vi "HapticSPM_force_bonding.vi"() -> ()   [LabVIEW 2023]
uses:
  Haptic-Programming-Interface/LabVIEW VIs/Haptic Prog Interface/Haptic Prog Interface.lvlib
panel:
  out "k":dbl format="%#_13g"
  out "Setpoint":dbl format="%#_13g"
  out "Force Function":string
  in  "Input Function":i32 min=0 max=4 step=1
  out "Potential vs Distance":cluster{dbl[], dbl[]}(graph)
  out "Force vs Distance":cluster{dbl[], dbl[]}(graph)
  out "Z-Position (pm)":dbl caption="Numeric" min=0.0 format="%#.1p"
  out "Force":dbl(knob) scale=-4.0..4.0
  in  "Gain":dbl=1.0 caption="Numeric" format="%.1g"
  # "Super Ultra Mega Haptic SPM Controller 3000"
  # "Height"
  # "Move pen in all three dimensions to calibrate before feeling surface\n\nClick \"ENTER\" to turn off recommended settings\n\nChange \"Setpoint\" and \"k\" parameters to adjust the feel of the force\n\nUse the \"PAGE UP\" or \"PAGE DOWN\" key to change the force function\n\nHold the pen as high as possible before changing force functions"
  # "Force"
  # "create bonding picture on this mod"
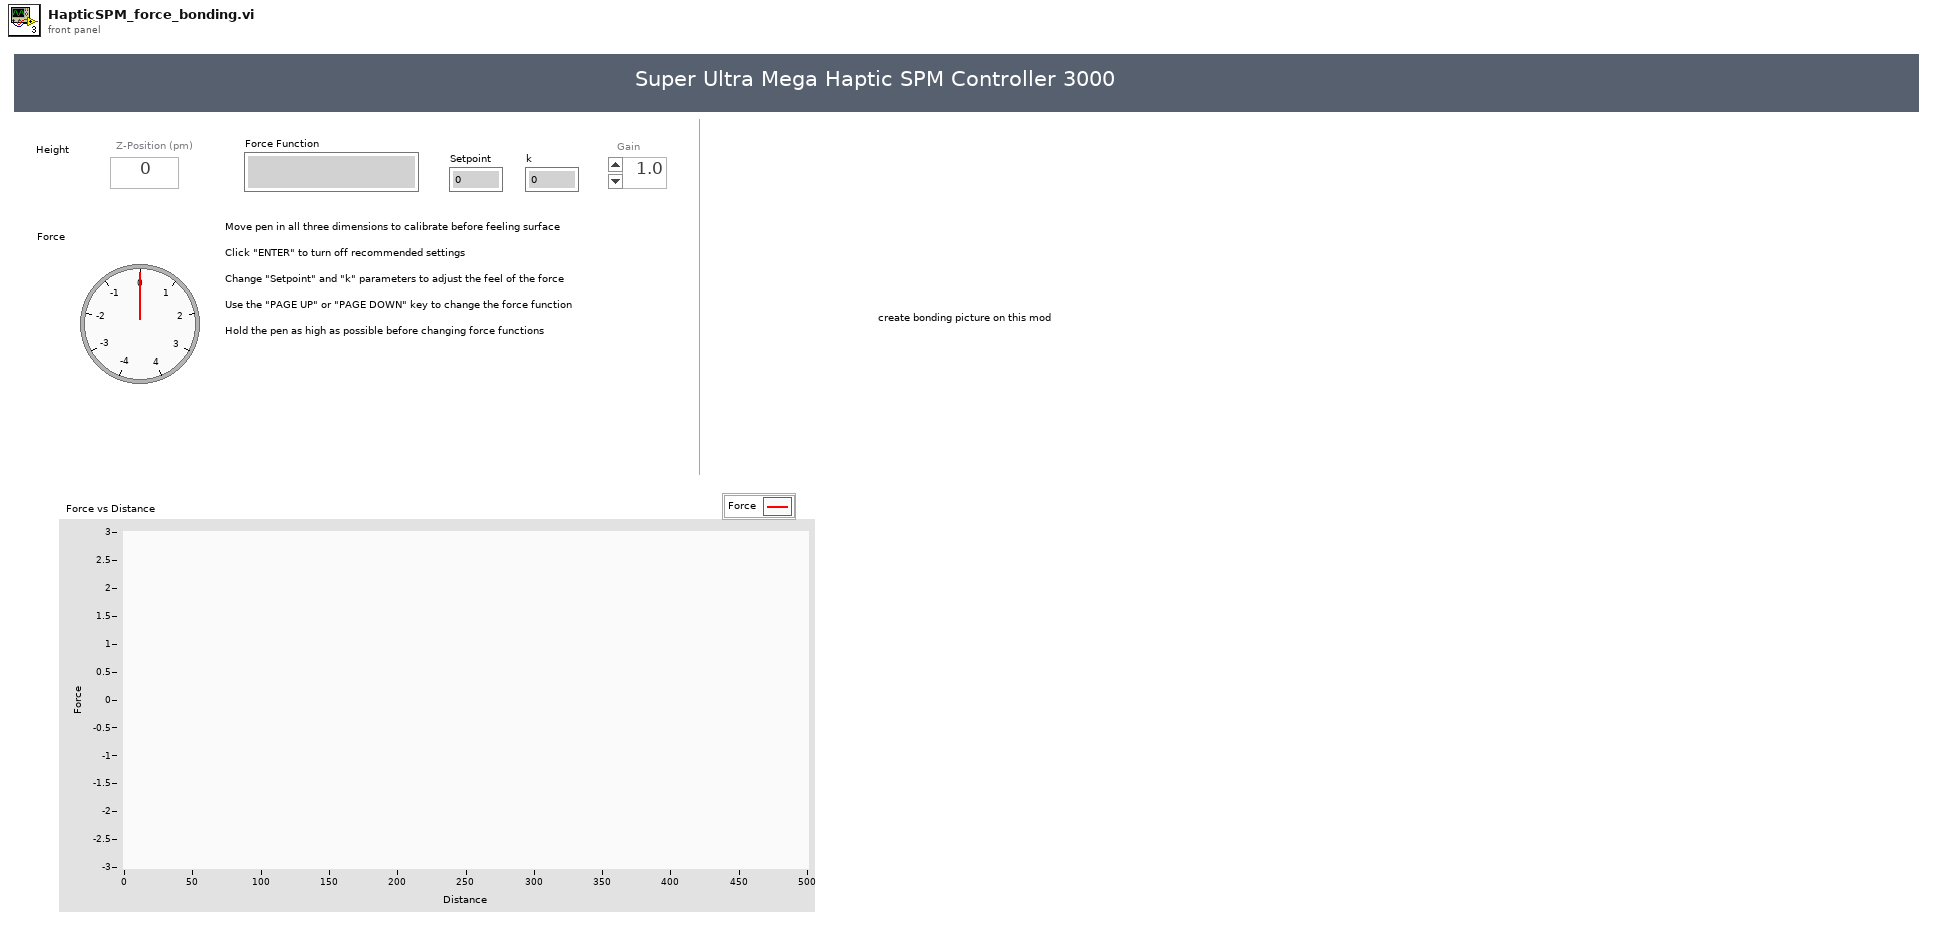
[diagram p1: front panel]
types:
  T1 = cluster{"Fx (N)":dbl, "Fy (N)":dbl, "Fz (N)":dbl}
  T2 = cluster{"kx (N/m)":dbl, "ky (N/m)":dbl, "kz (N/m)":dbl}
  T3 = cluster{"X Drag":bool, "Y Drag":bool, "Z Drag":bool}
  T4 = cluster{"x (mm)":dbl, "y (mm)":dbl, "z (mm)":dbl}
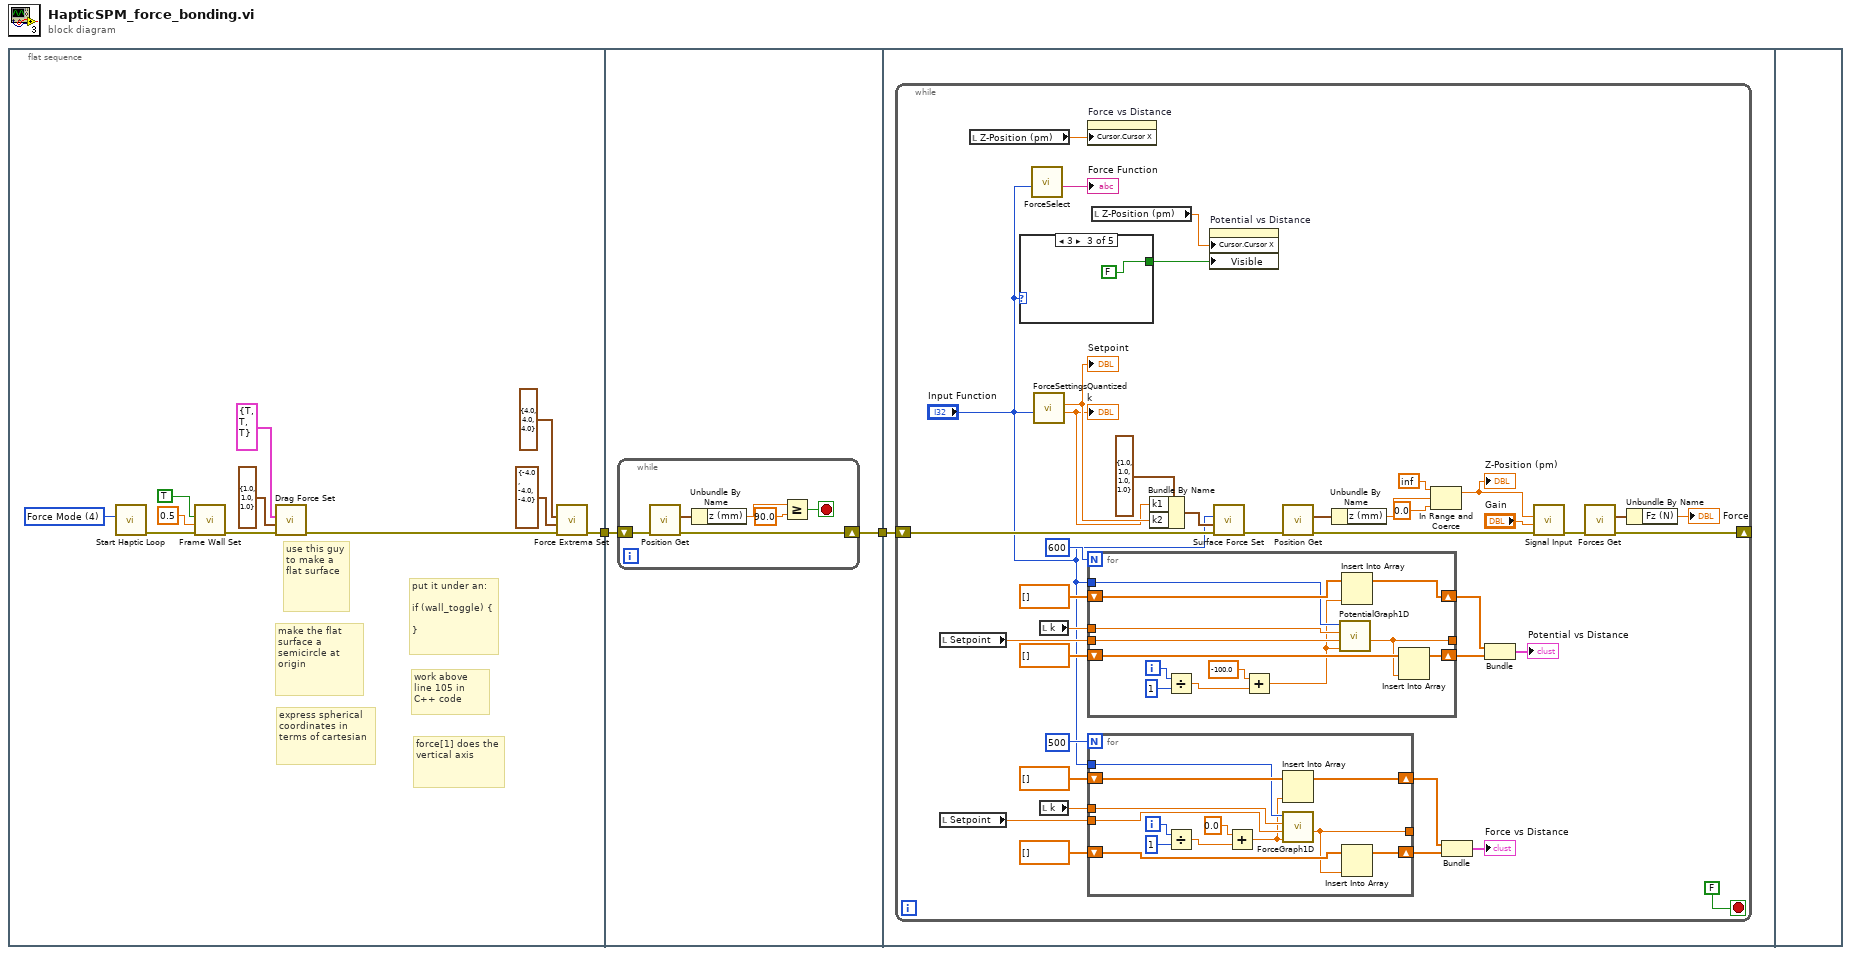
[diagram p0: block diagram]
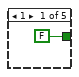
[diagram p2: hidden frame]
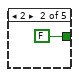
[diagram p3: hidden frame]
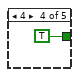
[diagram p4: hidden frame]
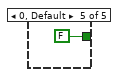
[diagram p5: hidden frame]
diagram:
  n1 = flat-sequence {
    tunnel: [w11] -> w2
    tunnel: w2 -> [w15]
    tunnel: [w14] -> w1
    tunnel: w1 -> [w22]
    frame #0 {
      w13 = u16 4 items=["Custom Mode", "Read Mode", "Write Mode", "Position Mode", "Force Mode"] ("Mode Selection")
      # "force[1] does the vertical axis"
      # "put it under an:\n\nif (wall_toggle) {\n\n}"
      # "work above line 105 in C++ code"
      # "express spherical coordinates in terms of cartesian"
      # "make the flat surface a semicircle at origin"
      # "use this guy to make a flat surface"
      n2 = call "Start Haptic Loop.vi"("Mode Selection"=w13) -> ("error out"=w4:errorcluster)  [unwired: 10 in]
      n3 = call "Frame Wall Set.vi"("error in (no error)"=w4, "Wall Stiffness (N/m)"=0.5 ("Wall Stiffness"), "Restrict to Frame"=TRUE) -> ("error out"=w3:errorcluster)  [unwired: 8 in]
      n4 = call "Drag Force Set.vi"("error in (no error)"=w3, "Drag Coefficients (N/m)"=T2 {"kx (N/m)"=1.0, "ky (N/m)"=1.0, "kz (N/m)"=1.0} ("Drag Coefficients"), "Drag Force Toggles"=T3 {"X Drag"=TRUE, "Y Drag"=TRUE, "Z Drag"=TRUE}) -> ("error out"=w12:errorcluster)  [unwired: 8 in]
      n5 = call "Force Extrema Set.vi"("error in (no error)"=w12, "Minimum Force (N)"=T1 {"Fx (N)"=-4.0, "Fy (N)"=-4.0, "Fz (N)"=-4.0} ("Minimum Force"), "Maximum Force (N)"=T1 {"Fx (N)"=4.0, "Fy (N)"=4.0, "Fz (N)"=4.0} ("Maximum Force")) -> ("error out"=w11:errorcluster)  [unwired: 8 in]
    }
    frame #1 {
      n6 = while {
        shift-right: [w20] -> w14
        shift-left: w15 -> [w21]
        stop <- w16 stop-if-true
        n7 = call "Position Get.vi"("error in (no error)"=w21) -> ("error out"=w20:errorcluster, "Position"=w19:T4)  [unwired: 9 in]
        n8 = Unbundle By Name(w19) -> ("z (mm)"=w18:dbl)
        n9 = Greater Or Equal?(x=w18, y=90.0) -> (x >= y?=w16:bool)
      }
    }
    frame #2 {
      n10 = while {
        shift-right: [w45] -> _
        shift-left: w22 -> [w61]
        stop <- FALSE ("Boolean") stop-if-true
        n11 = local read "Setpoint"() -> (w36:dbl)
        n12 = local read "Setpoint"() -> (w47:dbl)
        n13 = local read "Z-Position (pm)"() -> (w46:dbl)
        n14 = case shown="3" "Input Function" {
          tunnel: [FALSE FALSE FALSE TRUE FALSE] -> w34
          frame 1 {
          }
          frame 2 {
          }
          frame 3 {
          }
          frame 4 {
          }
          frame 0, Default {
          }
        }
        n15 = call "ForceSelect.vi"("Input Function"="Input Function") -> ("Force Function"=→"Force Function":string)  [unwired: 10 in]
        n16 = call "ForceSettingsQuantized.vi"("Function"="Input Function") -> ("k"=w23:dbl, "Setpoint"=w24:dbl)  [unwired: 9 in]
        "Setpoint" <- w24
        "k" <- w23
        n17 = local read "k"() -> (w37:dbl)
        n18 = local read "k"() -> (w48:dbl)
        n19 = property on="Force vs Distance" class="XYGraph (strict)"("Cursor.Cursor X"=w46) -> ()  [unwired: 2 in, 2 out]
        n20 = for {
          N: 600 -> [_]
          shift-right: [w79] -> w42
          shift-left: dbl[] [] -> [w77]
          shift-right: [w78] -> w43
          shift-left: dbl[] [] -> [w76]
          tunnel: "Input Function" -> [w72]
          tunnel: [w75] -> _
          tunnel: w36 -> [w74]
          tunnel: w37 -> [w73]
          i -> [w70]
          n21 = Divide(x=w70, y=1) -> (x/y=w69:dbl)
          n22 = Add(x=-100.0, y=w69) -> (x+y=w67:dbl)
          n23 = call "PotentialGraph1D.vi"("number"=w67, "Setpoint"=w74, "k"=w73, "Function"=w72) -> ("potential"=w75:dbl)  [unwired: 7 in]
          n24 = Insert Into Array(array=w76, new element=w67) -> (w78:dbl[])  [unwired: 1 in]
          n25 = Insert Into Array(array=w77, new element=w75) -> (w79:dbl[])  [unwired: 1 in]
        }
        n26 = for {
          N: 500 -> [_]
          shift-right: [w92] -> w53
          shift-left: dbl[] [] -> [w90]
          shift-right: [w91] -> w54
          shift-left: dbl[] [] -> [w89]
          tunnel: "Input Function" -> [w85]
          tunnel: [w88] -> _
          tunnel: w47 -> [w87]
          tunnel: w48 -> [w86]
          i -> [w83]
          n27 = Divide(x=w83, y=1) -> (x/y=w82:dbl)
          n28 = Add(x=0.0, y=w82) -> (x+y=w80:dbl)
          n29 = Insert Into Array(array=w89, new element=w80) -> (w91:dbl[])  [unwired: 1 in]
          n30 = call "ForceGraph1D.vi"("number"=w80, "Setpoint"=w87, "k"=w86, "Function"=w85) -> ("force"=w88:dbl)  [unwired: 7 in]
          n31 = Insert Into Array(array=w90, new element=w88) -> (w92:dbl[])  [unwired: 1 in]
        }
        n32 = local read "Z-Position (pm)"() -> (w35:dbl)
        n33 = Bundle By Name(cluster=cluster{"k1":dbl, "k2":dbl, "k3":dbl, "k4":dbl} {"k1"=1.0, "k2"=1.0, "k3"=1.0, "k4"=1.0} ("Force Constants"), "k1"=w23, "k2"=w24) -> (w57:cluster{"k1":dbl, "k2":dbl, "k3":dbl, "k4":dbl})
        n34 = property on="Potential vs Distance" class="XYGraph (strict)"("Cursor.Cursor X"=w35, "Visible"=w34) -> ()  [unwired: 2 in, 2 out]
        n35 = call "Surface Force Set.vi"("error in (no error)"=w61, "Force Constants"=w57, "Force Settings"="Input Function") -> ("error out"=w31:errorcluster)  [unwired: 8 in]
        n36 = call "Position Get.vi"("error in (no error)"=w31) -> ("error out"=w30:errorcluster, "Position"=w29:T4)  [unwired: 9 in]
        n37 = Unbundle By Name(w29) -> ("z (mm)"=w28:dbl)
        n38 = In Range and Coerce(upper limit=inf, x=w28, lower limit=0.0) -> (coerced(x)=w26:dbl)  [unwired: 1 out]
        "Z-Position (pm)" <- w26
        n39 = Bundle(w54, w53) -> (→"Force vs Distance":cluster{dbl[], dbl[]})  [unwired: 1 in]
        n40 = Bundle(w43, w42) -> (→"Potential vs Distance":cluster{dbl[], dbl[]})  [unwired: 1 in]
        n41 = call "Signal Input.vi"("error in (no error)"=w30, "Gain"="Gain", "Signal"=w26) -> ("error out"=w60:errorcluster)  [unwired: 8 in]
        n42 = call "Forces Get.vi"("error in (no error)"=w60) -> ("error out"=w45:errorcluster, "Force (N)"=w56:T1)  [unwired: 9 in]
        n43 = Unbundle By Name(w56) -> ("Fz (N)"=→"Force":dbl)
      }
    }
    frame #3 {
    }
  }
